vi "Real Determinant.vi"(2 "matrix type":T1(ring), 3 "Input Matrix":T2) -> (0 "error":i32, 1 "determinant":dbl format="%.2e")   [LabVIEW 2014, in "NI_AALBase.lvlib"]
doc: "Computes the <B>determinant</B> of <B>Input Matrix</B>. Wire data to the <B>Input Matrix</B> input to determine the polymorphic instance to use or manually select the instance."
uses:
  NI_AALBase.lvlib
  RealMatrix.ctl
  lvanlys.dll
  NI_Matrix.lvlib
panel:
  # "Determinant"
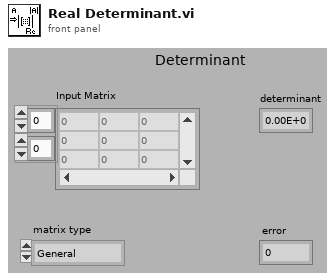
[diagram p1: front panel]
types:
  T1 = enum32{"General", "Positive Definite", "Lower Triangular", "Upper Triangular"}
  T2 = typedef "NI_Matrix.lvlib/RealMatrix.ctl" = dbl[][]
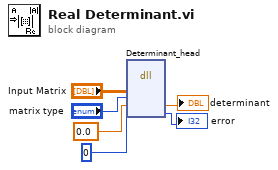
[diagram p0: block diagram]
diagram:
  n1 = dll-call lib="C:/Program Files (x86)/National Instruments/LabVIEW 2014/resource/lvanlys.*" fn="Determinant_head"("Input Matrix"="Input Matrix", "matrix type"="matrix type", 0.0, 0) -> (→"determinant":dbl, →"error":i32)  [unwired: 6 in, 2 out]
